vi "TSM DMM Read.vi"(0 "DMM TSM In":T1, 11 "error in":errorcluster) -> (4 "DMM TSM Out":T1, 6 "measurement":dbl[](array[numeric]), 15 "error out":errorcluster)   [LabVIEW 2019]
doc: "Use this VI to read the measurement from NI-DMM instruments in the pin map associated with the test program."
uses:
  Pin Map/TSM DMM.ctl
  <vilib>/NI_TestStand_SemiconductorModule/NI_TestStand_Semiconductor_Module.lvlibp/PinMap/PinQueryContext/MultiplePinMultipleSessionQueryContext/MultiplePinMultipleSessionQueryContext.lvclass
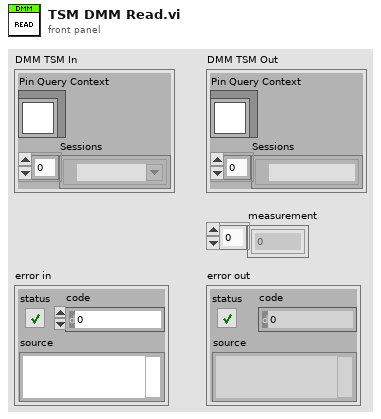
[diagram p1: front panel]
types:
  T1 = typedef "TSM DMM.ctl" = cluster{"Pin Query Context":refnum<class "MultiplePinMultipleSessionQueryContext.lvclass">, "Sessions":refnum<k15>[]}
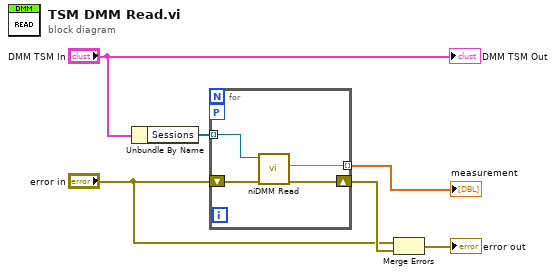
[diagram p0: block diagram]
diagram:
  n1 = Unbundle By Name("DMM TSM In") -> ("Sessions"=w2:refnum<k15>[])
  n2 = for {
    workers-P: _ -> [_]
    tunnel: [w8] -> w3 mode=indexing
    tunnel: w2 -> [w7] mode=indexing
    shift-right: [w9] -> w6
    shift-left: "error in" -> [w10]
    n3 = call <instrlib>:"niDMM Read.vi"("error in (no error)"=w10, "instrument handle"=w7) -> ("error out"=w9:errorcluster, "Measurement"=w8:dbl)  [unwired: 7 in, 1 out]
  }
  "measurement" <- w3
  n4 = Merge Errors("error in", w6) -> (→"error out":errorcluster)
  "DMM TSM Out" <- "DMM TSM In"
